vi "Power OFF-Single.vi"(8 "error in (no error)":errorcluster, 11 "Resource name":string) -> (0 "error out":errorcluster, 3 "Status":string)   [LabVIEW 2021]
doc: "This VI will reset the source and load devices, which results in powering off the DUT for single-channel configuration."
uses:
  <instrlib>/niDCPower/nidcpower.llb/niDCPower Get Channel Name From String.vi
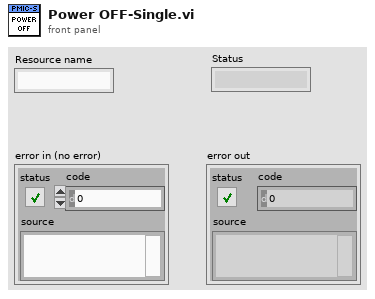
[diagram p1: front panel]
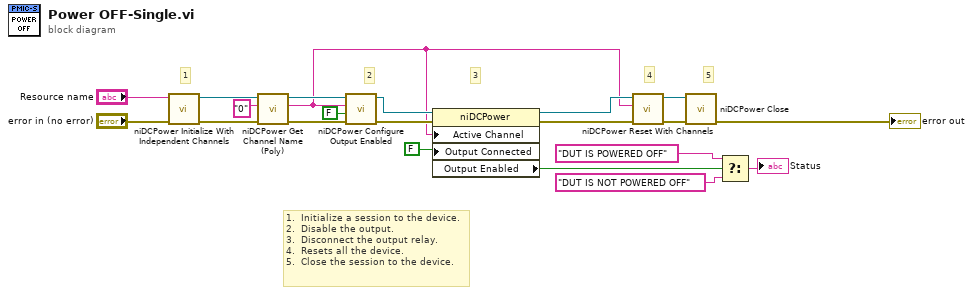
[diagram p0: block diagram]
diagram:
  # "5"
  # "4"
  # "3"
  # "2"
  # "1"
  # "1.  Initialize a session to the device.\n2.  Disable the output.\n3.  Disconnect the output relay.\n4.  Resets all the device.\n5.  Close the session to the device."
  n1 = call <instrlib>:"niDCPower Initialize With Independent Channels.vi"("error in (no error)"="error in (no error)", "resource name"="Resource name") -> ("error out"=w19:errorcluster, "instrument handle out"=w21:refnum<k15>)  [unwired: 8 in]
  n2 = call-poly <instrlib>:"niDCPower Get Channel Name (Poly).vi"("error in (no error)"=w19, "index"="0", "instrument handle"=w21) -> ("error out"=w15:errorcluster, "name"=w7:string, "instrument handle out"=w17:refnum<k15>)  [unwired: 6 in]
  n3 = call <instrlib>:"niDCPower Configure Output Enabled.vi"("error in (no error)"=w15, "output enabled"=FALSE, "channel name"=w7, "instrument handle"=w17) -> ("error out"=w11:errorcluster, "instrument handle out"=w9:refnum<k15>)  [unwired: 6 in]
  n4 = property class="niDCPower"(reference=w9, error in=w11, "Active Channel"=w7, "Output Connected"=FALSE ("Source:Output Connected")) -> (reference out=w8:refnum<k15>, error out=w10:errorcluster, "Output Enabled"=w4:bool)
  n5 = call <instrlib>:"niDCPower Reset With Channels.vi"("error in (no error)"=w10, "channel name"=w7, "instrument handle"=w8) -> ("error out"=w14:errorcluster, "instrument handle out"=w13:refnum<k15>)  [unwired: 7 in]
  n6 = call <instrlib>:"niDCPower Close.vi"("error in (no error)"=w14, "instrument handle"=w13) -> ("error out"=→"error out":errorcluster)  [unwired: 9 out]
  n7 = Select(t="DUT IS POWERED OFF" ("Status"), s=w4, f="DUT IS NOT POWERED OFF") -> (s? t:f=→"Status":string)
